vi "One Element Stream.vi"() -> ()   [LabVIEW 2023]
doc: "This VI demonstrates basic use of the One Element Stream, a channel wire that communicates data between two parallel loops and easily handling many of the complex scenarios for managing the controlled shutdown of that connection."
uses:
  <extravilib>/ChannelInstances/One Element Stream-i32/Instantiate.vi
  <extravilib>/ChannelInstances/One Element Stream-i32/EndpointRead.vi
  <extravilib>/ChannelInstances/One Element Stream-i32/Endpoint.vi
  <extravilib>/ChannelInstances/One Element Stream-i32.lvlib
panel:
  in  "Consumer Stop Value":i32=-1
  in  "Emergency Stop Producer":bool
  out "Data Consumed":i32(graph)
  out "Data Produced":i32(graph)
  in  "Stop Consumer":bool
  in  "Stop Producer":bool
  # "Overview: Demonstrates how to use the One Element Stream, which is one of the channel wire templates that ships with LabVIEW.  One Element Streams are restricted to a single writer and a single reader to provide point-to-point communication. The One Element Stream provides control for a wide variation in communication needs. This example shows how signals raised from different parts of the program can be easily transmitted to the rest of the application. \n\nInstructions:\n1. Run the VI. Press the Normal Stop Producer button to see the producer stop and the consumer continue until it catches up. This is a normal stop generated from the producer.\n2. Run the VI again. Press the Emergency Stop Producer button to see both stop at the same time. This is an emergency stop generated from the producer.\n3. Run the VI again. Press the Stop Consumer button to see both stop at the same time. This is an emergency stop generated from the consumer.\n4. Run the VI again. Change the Consumer Stop Value to a value between 0 and 9 to see both loops stop as soon as the consumer receives that value. This is another example of an emergency stop generated from the consumer."
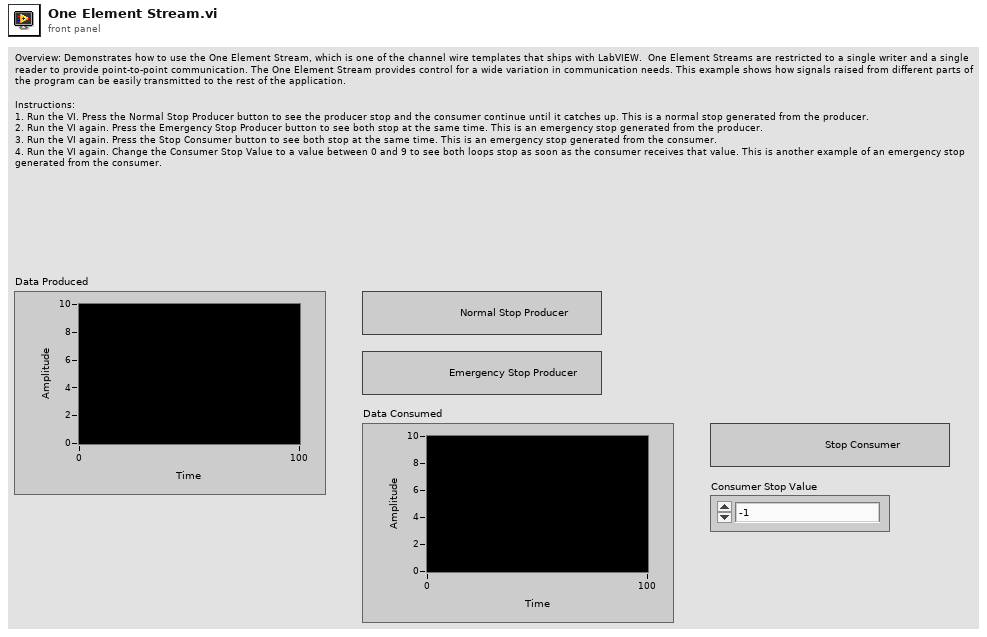
[diagram p1: front panel]
types:
  T1 = typedef "One Element Stream-i32.lvlib/)Channel.ctl" = refnum<queue>
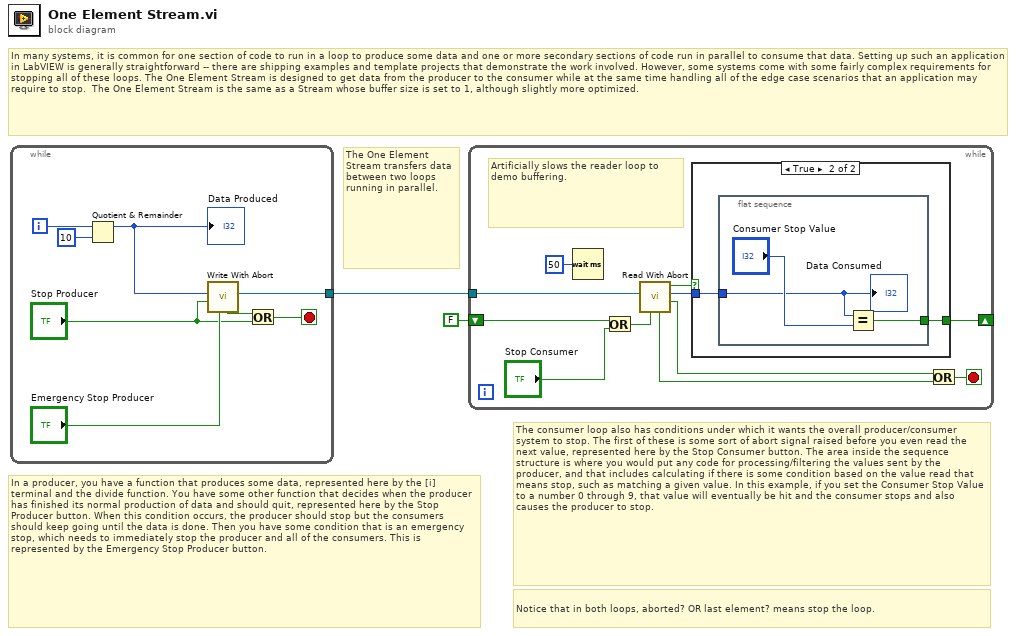
[diagram p0: block diagram]
diagram:
  # "Notice that in both loops, aborted? OR last element? means stop the loop."
  # "The consumer loop also has conditions under which it wants the overall producer/consumer system to stop. The first of these is some sort of abort signal raised before you even read the next value, represented here by the Stop Consumer button. The area inside the sequence structure is where you would put any code for processing/filtering the values sent by the producer, and that includes calculating if there is some condition based on the value read that means stop, such as matching a given value. In this example, if you set the Consumer Stop Value to a number 0 through 9, that value will eventually be hit and the consumer stops and also causes the producer to stop."
  # "The One Element Stream transfers data between two loops running in parallel."
  # "In a producer, you have a function that produces some data, represented here by the [i] terminal and the divide function. You have some other function that decides when the producer has finished its normal production of data and should quit, represented here by the Stop Producer button. When this condition occurs, the producer should stop but the consumers should keep going until the data is done. Then you have some condition that is an emergency stop, which needs to immediately stop the producer and all of the consumers. This is represented by the Emergency Stop Producer button."
  # "In many systems, it is common for one section of code to run in a loop to produce some data and one or more secondary sections of code run in parallel to consume that data. Setting up such an application in LabVIEW is generally straightforward -- there are shipping examples and template projects that demonstrate the work involved. However, some systems come with some fairly complex requirements for stopping all of these loops. The One Element Stream is designed to get data from the producer to the consumer while at the same time handling all of the edge case scenarios that an application may require to stop.  The One Element Stream is the same as a Stream whose buffer size is set to 1, although slightly more optimized."
  n1 = while {
    tunnel: [w6] -> w2
    i -> [w9]
    stop <- w3 stop-if-true
    n2 = Quotient & Remainder(x=w9, y=10) -> (x-y*floor(x/y)=w8:i32)  [unwired: 1 out]
    "Data Produced" <- w8
    n3 = call <extravilib>:"Write With Abort.vi"("abort"="Emergency Stop Producer", "last element? (F)"="Stop Producer", "element"=w8) -> ("channel"=w6:T1, "aborted?"=w5:bool)  [unwired: 6 in, 1 out]
    n4 = Or(x=w5, y="Stop Producer") -> (x .or. y?=w3:bool)
  }
  n5 = while {
    tunnel: w2 -> [w21]
    shift-right: [w14] -> _
    shift-left: FALSE -> [w13]
    stop <- w20 stop-if-true
    # "Artificially slows the reader loop to demo buffering."
    n6 = Wait (ms)(milliseconds to wait=u32 50) -> ()  [unwired: 1 out]
    n7 = Or(x=w13, y="Stop Consumer") -> (x .or. y?=w11:bool)
    n8 = call <extravilib>:"Read With Abort.vi"("abort"=w11, "channel"=w21) -> ("last element?"=w16:bool, "element"=w18:i32, "element valid?"=w17:bool, "aborted?"=w15:bool)  [unwired: 5 in, 1 out]
    n9 = case shown="True" w17 {
      tunnel: w18 -> [_ w23]
      tunnel: [_ w22] -> w14
      frame False {
      }
      frame True {
        n10 = flat-sequence {
          tunnel: w23 -> [w25]
          tunnel: [w24] -> w22
          frame #0 {
            n11 = Equal?(x=w25, y="Consumer Stop Value") -> (x = y?=w24:bool)
            "Data Consumed" <- w25
          }
        }
      }
    }
    n12 = Or(x=w16, y=w15) -> (x .or. y?=w20:bool)
  }
